vi "Post-Install Custom Action.vi"(10 "Variant":variant) -> (0 "error out":errorcluster)   [LabVIEW 2019]
doc: "Opens the Quick Drop Panel and Diagram Shortcuts VI to replace the LabVIEW.ini keys with Ryan's Shortcuts."
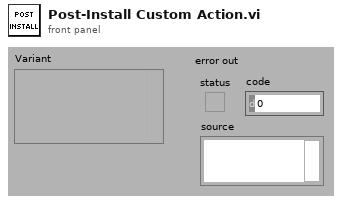
[diagram p1: front panel]
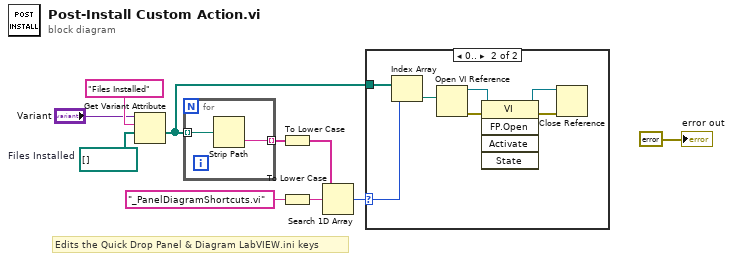
[diagram p0: block diagram]
diagram:
  w7 = path[] []  # Files Installed
  # "Edits the Quick Drop Panel & Diagram LabVIEW.ini keys"
  n1 = Get Variant Attribute(Variant="Variant", name="Files Installed", default value (empty Variant)=w7) -> (value=w1:path[])  [unwired: 1 in, 3 out]
  n2 = for {
    tunnel: w1 -> [w12] mode=indexing
    tunnel: [w11] -> w6 mode=indexing
    n3 = Strip Path(path=w12) -> (name=w11:string)  [unwired: 1 out]
  }
  n4 = To Lower Case(string=w6) -> (all lower case string=w5:string[])
  n5 = To Lower Case(string="_PanelDiagramShortcuts.vi" ("element")) -> (all lower case string=w3:string)
  n6 = Search 1D Array(1D array=w5, element=w3) -> (index of element=w2:i32)  [unwired: 1 in]
  n7 = case shown="0.." w2 {
    selector: w2 -> [_ w19]
    tunnel: w1 -> [_ w18]
    frame ..-1 {
    }
    frame 0.. {
      n8 = Index Array(array=w18, index=w19) -> (element=w17:path)
      n9 = Open VI Reference(vi path=w17) -> (vi reference=w16:refnum<vi>, error out=w15:errorcluster)  [unwired: 5 in]
      n10 = invoke class="VI" method="FP.Open"(reference=w16, error in=w15) -> (reference out=w13:refnum<vi>, error out=w14:errorcluster)  [unwired: 3 in, 3 out]
      n11 = Close Reference(reference=w13, error in (no error)=w14) -> ()  [unwired: 1 out]
    }
  }
  "error out" <- errorcluster {"status"=FALSE, "code"=0, "source"=""} ("error out")
